vi "Scale ADXL345 Data.vi"(11 "Raw":i16) -> (3 "Scaled":fxp<+/-,14,4>)   [LabVIEW 2015]
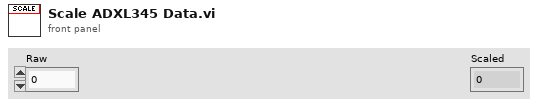
[diagram p1: front panel]
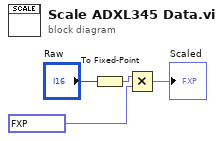
[diagram p0: block diagram]
diagram:
  n1 = To Fixed-Point(number="Raw") -> (fixed-point=w4:fxp<+/-,10,10>)  [unwired: 1 in]
  n2 = Multiply(x=w4, y=fxp<+/-,14,1> 0.0078125) -> (x*y=→"Scaled":fxp<+/-,14,4>)
